vi "Add Virtual Instrument.vi"(6 "<JSON CFG>":string, 8 "Error In":errorcluster, 11 "reference in":refnum<class "Measure and Stimulus Subsystems.lvclass">) -> (0 "Error Out":errorcluster, 3 "reference out":refnum<class "Measure and Stimulus Subsystems.lvclass">)   [LabVIEW 2023, in "HAL GOOP4.lvlib" / "Measure and Stimulus Subsystems.lvclass"]
uses:
  Measure and Stimulus Subsystems.lvclass
  Virt Instrument Base/Virt Instr Base.lvclass
  <vilib>/Utility/miscctls.llb/LVMapReplaceAction.ctl
  580f934a-731d-4e43-beb4-3f6aa3408910.vi
  <vilib>/JDP Science/JSONtext/Find Item.vi
  <vilib>/JDP Science/JSONtext/Next JSON Value.vi
  <vilib>/JDP Science/JSONtext/String Subset.vi
  <vilib>/JDP Science/JSONtext/Parsing/Advance past next JSON Value (inlined COPY).vi
  <vilib>/JDP Science/JSONtext/Parsing/Advance past whitespace.vi
  <vilib>/JDP Science/JSONtext/Parsing/Advance past String.vi
  <vilib>/JDP Science/JSONtext/Parsing/Advance past Number.vi
  <vilib>/JDP Science/JSONtext/Parsing/Advance past Line Ending.vi
  <vilib>/JDP Science/JSONtext/Parsing/Parse Full Path or Item Name.vi
  <vilib>/JDP Science/JSONtext/Parsing/Advance past Array.vi
  <vilib>/JDP Science/JSONtext/Parsing/Advance past Object.vi
  <vilib>/JDP Science/JSONtext/support/Error Cluster From Code.vi
  <vilib>/JDP Science/JSONtext/Offset/Find Item Locations by Path.vi
  <vilib>/JDP Science/JSONtext/JSON text to Variant.vi
  <vilib>/Utility/error.llb/Error Cluster From Error Code.vi
  <vilib>/JDP Science/JSONtext/LVClass Serializer/JSONtext LVClass Serializer.lvclass
  <vilib>/ErrorRing/Error Ring.xnode
  Measure and Stimulus Subsystems.lvclass/Measure and Stimulus Subsystems.ctl
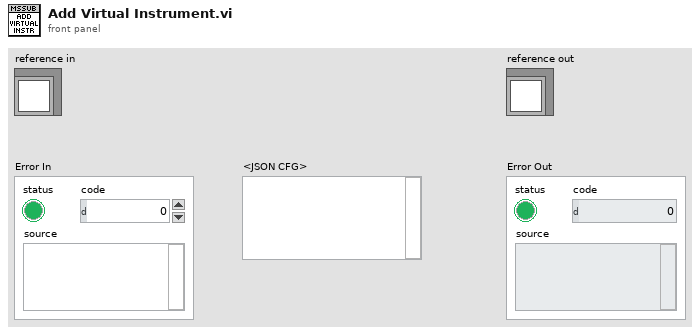
[diagram p1: front panel]
types:
  T1 = typedef "LVMapReplaceAction.ctl" = enum32{"Modify Entry only if found", "Add or Modify Entry", "Delete Entry"}
  T2 = cluster{"Target Ident":string, "Instr Ident":string, "Const Action Data":string, "Class":string}[]
  T3 = typedef "HAL GOOP4.lvlib/Measure and Stimulus Subsystems.lvclass/ObjectAttributes.ctl" = cluster{"Virt Instr":map{string, refnum<class "Virt Instr Base.lvclass">}, "Phys Instr":map{string, cluster{"Instrument Base":refnum<class "Instr Base.lvclass">, "Ref Count":u8}}}
  T4 = map{string, refnum<class "Virt Instr Base.lvclass">}
  T5 = map{string, cluster{"Instrument Base":refnum<class "Instr Base.lvclass">, "Ref Count":u8}}
  T6 = cluster{"Instrument Base":refnum<class "Instr Base.lvclass">, "Ref Count":u8}
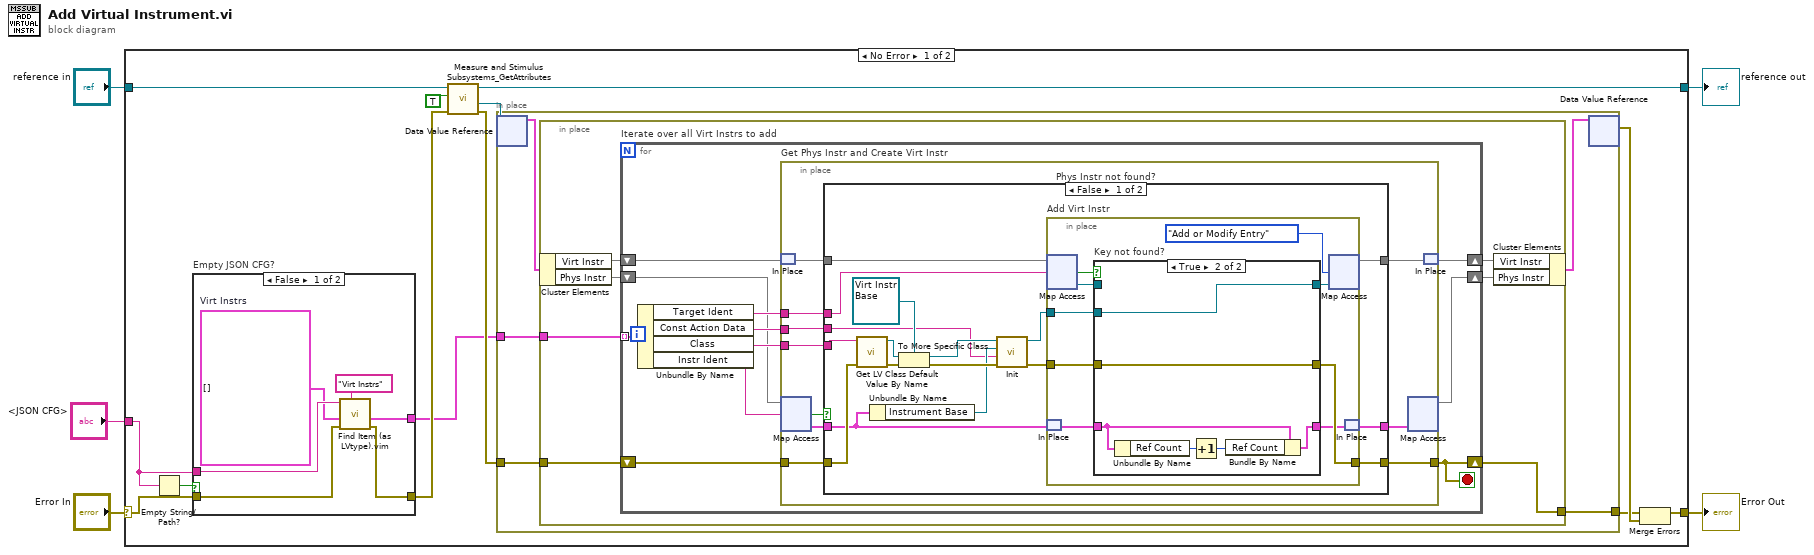
[diagram p0: block diagram]
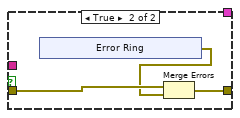
[diagram p2: hidden frame]
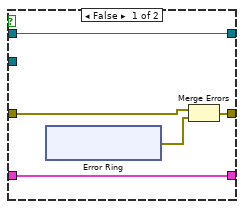
[diagram p3: hidden frame]
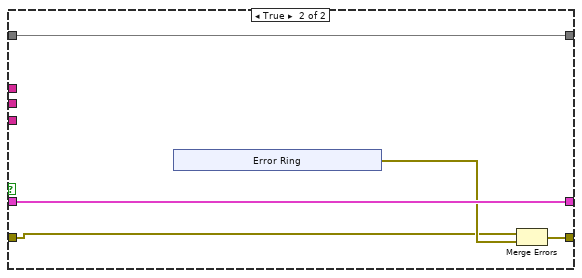
[diagram p4: hidden frame]
diagram:
  n1 = case shown="No Error" "Error In" {
    selector: "Error In" -> [w8 w119]
    tunnel: [w15 w119] -> w4
    tunnel: [w16 w118] -> w2
    tunnel: "reference in" -> [w18 w118]
    tunnel: "<JSON CFG>" -> [w6 _]
    frame No Error {
      n2 = Empty String/Path?(string/path=w6) -> (empty?=w7:bool)
      n3 = case "Empty JSON CFG?" shown="False" w7 {
        tunnel: w8 -> [w24 w27]
        tunnel: [w22 w25] -> w10
        tunnel: w6 -> [w23 _]
        tunnel: [w19 _] -> w9
        frame False {
          w21 = T2 []  # Virt Instrs
          n4 = call "Find Item (as LVtype).vim"("$Path or Item Name"="Virt Instrs", "error in (no error)"=w24, "Data Type and Default Value"=w21, "JSON"=w23) -> ("error out"=w22:errorcluster, "Data"=w19:T2)  [unwired: 4 in, 2 out]
        }
        frame True {
          n5 = xnode "Error Ring"() -> ("error out"=w26:errorcluster)
          n6 = Merge Errors(w27, w26) -> (w25:errorcluster)
        }
      }
      n7 = call "Measure and Stimulus Subsystems_GetAttributes.vi"("Error In"=w10, "OnlyGetDvrReference(False)"=TRUE, "reference in"=w18) -> ("Error Out"=w12:errorcluster, "DataRef"=w14:refnum<data-value>, "reference out"=w16:refnum<class "Measure and Stimulus Subsystems.lvclass">)  [unwired: 5 in, 1 out]
      n8 = in-place {
        in-place-border: w12 -> [w37]
        in-place-border: [w36] -> w11
        in-place-border: w9 -> [w35]
        n9 = in-place-dvr #1(w14) -> (w34:T3)  [unwired: 1 out]
        n10 = in-place {
          in-place-border: w37 -> [w44]
          in-place-border: [w43] -> w36
          in-place-border: w35 -> [w42]
          n11 = in-place-cluster #2(w34) -> ("Virt Instr"=w40:T4, "Phys Instr"=w41:T5)
          n12 = for "Iterate over all Virt Instrs to add" {
            tunnel: w42 -> [w55] mode=indexing
            shift-right: [w51] -> w43
            shift-left: w44 -> [w53]
            shift-right: [w46] -> w38
            shift-left: w41 -> [w49]
            shift-right: [w47] -> w39
            shift-left: w40 -> [w48]
            stop <- w51 stop-if-true
            n13 = Unbundle By Name(w55) -> ("Target Ident"=w50:string, "Const Action Data"=w52:string, "Class"=w54:string, "Instr Ident"=w45:string)
            n14 = in-place "Get Phys Instr and Create Virt Instr" {
              in-place-border: w54 -> [w65]
              in-place-border: w53 -> [w64]
              in-place-border: w52 -> [w63]
              in-place-border: [w62] -> w51
              in-place-border: w50 -> [w61]
              n15 = in-place-match #3(w48) -> (w60:T4)
              n16 = in-place-map #4(w49, w45) -> (w58:T6, w56:bool)  [unwired: 1 in]
              n17 = case "Phys Instr not found?" shown="False" w56 {
                tunnel: w65 -> [w82 _]
                tunnel: w64 -> [w81 w108]
                tunnel: w63 -> [w66 _]
                tunnel: [w76 w112] -> w62
                tunnel: w61 -> [w75 _]
                tunnel: w60 -> [w70 w110]
                tunnel: [w69 w110] -> w59
                tunnel: w58 -> [w68 w111]
                tunnel: [w67 w111] -> w57
                frame False {
                  n18 = call <vilib>:"Get LV Class Default Value By Name.vi"("error in (no error)"=w81, "class name"=w82) -> ("error out"=w80:errorcluster, "object"=w78:refnum<class>)  [unwired: 8 in]
                  n19 = Unbundle By Name(w68) -> ("Instrument Base"=w71:refnum<class "Instr Base.lvclass">)
                  n20 = To More Specific Class(target class=refnum<class "Virt Instr Base.lvclass"> refnum ("HAL GOOP4.lvlib:Virtual Instrument Base.lvclass"), reference=w78, error in=w80) -> (specific class reference=w73:refnum<class "Virt Instr Base.lvclass">, error out=w77:errorcluster)
                  n21 = call-dynamic "Init.vi"("error in (no error)"=w77, "Constant Action Data"=w66, "HAL GOOP4.lvlib:Instrument Base"=w71, "Virt Instrument Base in"=w73) -> ("error out"=w74:errorcluster, "Virt Instrument Base out"=w72:refnum<class "Virt Instr Base.lvclass">)  [unwired: 6 in]
                  n22 = in-place "Add Virt Instr" {
                    in-place-border: w72 -> [w89]
                    in-place-border: w74 -> [w87]
                    in-place-border: [w86] -> w76
                    n23 = in-place-map #5(w70, w75) -> (w90:refnum<class "Virt Instr Base.lvclass">, w91:bool)  [unwired: 1 in]
                    n24 = in-place-match #6(w68) -> (w84:T6)
                    n25 = case "Key not found?" shown="True" w91 {
                      tunnel: w90 -> [w93 _]
                      tunnel: w89 -> [_ w102]
                      tunnel: [w93 w102] -> w88
                      tunnel: w87 -> [w96 w107]
                      tunnel: [w94 w107] -> w86
                      tunnel: w84 -> [w92 w104]
                      tunnel: [w92 w103] -> w83
                      frame False {
                        n26 = xnode "Error Ring"() -> ("error out"=w95:errorcluster)
                        n27 = Merge Errors(w96, w95) -> (w94:errorcluster)
                      }
                      frame True {
                        n28 = Unbundle By Name(w104) -> ("Ref Count"=w106:u8)
                        n29 = Increment(x=w106) -> (x+1=w105:u8)
                        n30 = Bundle By Name(cluster=w104, "Ref Count"=w105) -> (w103:T6)
                      }
                    }
                    n31 = in-place-map #5(w88, LVMapReplaceAction."Add or Modify Entry" ("action")) -> (w69:T4)  [unwired: 2 out]
                    n32 = in-place-match #6(w83) -> (w67:T6)
                  }
                }
                frame True {
                  n33 = xnode "Error Ring"() -> ("error out"=w109:errorcluster)
                  n34 = Merge Errors(w108, w109) -> (w112:errorcluster)
                }
              }
              n35 = in-place-map #4(w57) -> (w46:T5)  [unwired: 1 in, 2 out]
              n36 = in-place-match #3(w59) -> (w47:T4)
            }
          }
          n37 = in-place-cluster #2("Virt Instr"=w39, "Phys Instr"=w38) -> (w33:T3)
        }
        n38 = in-place-dvr #1(w33) -> (w17:errorcluster)  [unwired: 1 out]
      }
      n39 = Merge Errors(w11, w17) -> (w15:errorcluster)
    }
    frame Error {
    }
  }
  "Error Out" <- w4
  "reference out" <- w2
